vi "Make Receiver.vi"(8 "error in (no error)":errorcluster, 11 "Coupled Message Rescripter in":refnum<class "Coupled Message Rescripter.lvclass">) -> (0 "error out":errorcluster, 3 "Coupled Message Rescripter out":refnum<class "Coupled Message Rescripter.lvclass">)   [LabVIEW 2020, in "Message Rescripter.lvlib" / "Coupled Message Rescripter.lvclass"]
uses:
  Coupled Message Rescripter.lvclass
  MessageMakerProvider/_Message Maker/_Maker Classes/Coupled Message Scripter/Coupled Message Scripter.lvclass
  MessageMakerProvider/_Message Maker/_Maker Classes/Message Scripter/Message Scripter.lvclass
  Message Rescripter.lvlib
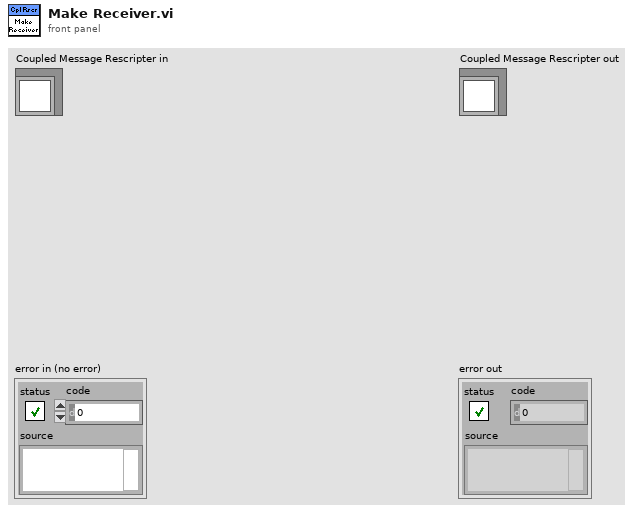
[diagram p1: front panel]
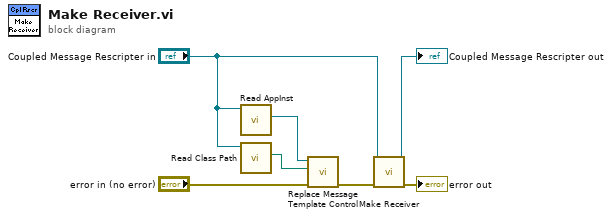
[diagram p0: block diagram]
diagram:
  n1 = call "Read AppInst.vi"("Message Maker in"="Coupled Message Rescripter in") -> ("AppInst"=w3:refnum<vi>)  [unwired: 10 in]
  n2 = call "Read Class Path.vi"("Message Scripter in"="Coupled Message Rescripter in") -> ("Class Path"=w4:path)  [unwired: 10 in]
  n3 = call "Replace Message Template Control.vi"("error in (no error)"="error in (no error)", "Class Path"=w4, "App Inst"=w3) -> ("error out"=w6:errorcluster)  [unwired: 8 in]
  n4 = call-parent "Make Receiver.vi"("error in (no error)"=w6, "Coupled Message Scripter in"="Coupled Message Rescripter in") -> ("error out"=→"error out":errorcluster, "Coupled Message Scripter out"=→"Coupled Message Rescripter out":refnum<class "Coupled Message Rescripter.lvclass">)  [unwired: 8 in]
